vi "D-O Module (Main).vi"(7 "Name of Parent Panel":string="Main.vi", 9 "New Center Coords":T1={"Horizontal"=470, "Vertical"=200}, 10 "Config":variant, 11 "Main UI Message Queue":refnum<queue>) -> ()   [LabVIEW 2018, in "D-O Module.lvlib"]
doc: "This Continuous Measurement sample project is based on the Queued Message Handler template.\n\nThe Event Handling Loop generates messages based on user interface actions.\n\nThe Message Handling Loop processes messages generated by the Event Handling Loop, or by other messages. There are also Acquisition and Logging message handling loop subVIs, and a chart updating loop."
uses:
  D-O Module.lvlib
  support/Message Queue/Message Cluster.ctl
  <vilib>/Utility/miscctls.llb/LVPoint32TypeDef.ctl
  controls/UI Data.ctl
  controls/UI State.ctl
  D-O Module State Cluster.ctl
  D-O Module Config Cluster.ctl
  Valve Clusters.ctl
  D-O Module Settings Cluster.ctl
  D-O Device Settings Cluster.ctl
  VICI Electronic Actuator/VICI Electronic Actuator Settings.ctl
  Measure Instrument/State Enum.ctl
  D-O Module Display.ctl
  Sequencing/Squence Update Cluster.ctl
  support/Message Queue/Enqueue Message (Single).vi
  support/User Event - Stop/User Event - Stop.lvlib
  support/Support Library.lvlib
  support/Message Queue/Message Queue.lvlib
  Measure Instrument/D-O Module Engine.lvlib
  Measure Instrument/Feed Module Engine.lvlib
  Sequencing/Sequencing Library.lvlib
  D-O Settings Dialog.vi
  support/Command Log VIs/Command Logging.lvlib
  DIO Valve/VICI Electronic Actuator.lvlib
  Report Generation/Report Generation.lvlib
panel:
  out "Sequence Started":bool
  in  "Settings Button":bool
  out "ScanCode":i16
  out "Ring":u16(ring)=2
  out "Log File path":path
  out "Status":string
  in  "Exit":bool
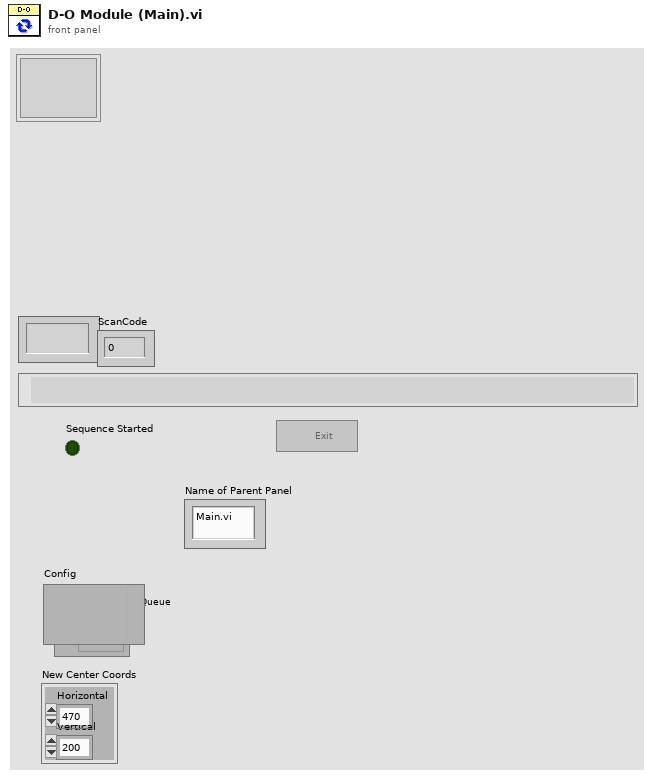
[diagram p1: front panel]
types:
  T1 = typedef "LVPoint32TypeDef.ctl" = cluster{"Horizontal":i32, "Vertical":i32}
  T2 = enum32{"Invalid", "Default", "Floating", "Floating/Auto-Hide", "Modal"}
  T3 = typedef "D-O Module.lvlib/D-O Module Config Cluster.ctl" = cluster{"GUID":string, "Drop Coords":T1, "Process Name":string, "User name":string, "Queue Name":string, "Settings":T4, "Load Count":i32}
  T4 = typedef "D-O Module.lvlib/Valve Clusters.ctl" = cluster{"Valve Settings":T5, "Valve Type":enum16{"Default", "Digital Output Valve", "VICI Electronic Actuator"}, "Time On (Sec)":dbl, "Time Off (Sec)":dbl, "Run?":bool}
  T5 = typedef "D-O Module.lvlib/D-O Module Settings Cluster.ctl" = cluster{"D-O Settings":T6, "VICI Electronic Actuator":T7}
  T6 = typedef "D-O Module.lvlib/D-O Device Settings Cluster.ctl" = cluster{"DAQmx Task Name":refnum<k21>, "Output Channel":u16, "Output Channel Names":string[]}
  T7 = typedef "VICI Electronic Actuator.lvlib/VICI Electronic Actuator Settings.ctl" = cluster{"VISA resource name":refnum<visa-resource-name>, "Mode":enum16{"Two Positions With Stops", "Two Positions Without Stops", "Mutiposition"}, "Simulated":bool}
  T8 = typedef "D-O Module.lvlib/D-O Module State Cluster.ctl" = cluster{"D-O Module Config":T3, "State":T9, "Start Time":timestamp, "Current Time":timestamp, "First Iteration":bool, "Data":cluster{"Valve State":T5}, "Process Name":string, "Queue Name":string, "Program On?":bool}
  T9 = typedef "Feed Module.lvlib/Feed Module Engine.lvlib/State Enum.ctl" = enum16{"Measuring", "Idle", "Paused"}
  T10 = typedef "UI State.ctl" = enum16{"Idle", "Acquiring and Logging", "Waiting for Exit", "Waiting for Exit (Acq Stopped)", "Waiting for Exit (Log Stopped)", "Waiting for Stop", "Waiting for Stop (Acq Stopped)", "Waiting for Stop (Log Stopped)"}
  T11 = typedef "UI Data.ctl" = cluster{"Start Ref":refnum<vi>, "Trigger Ref":refnum<vi>, "Stop Ref":refnum<vi>, "Settings Ref":refnum<vi>, "Status Ref":refnum<vi>, "Exit Ref":refnum<vi>, "Data Ref":refnum<vi>}
  T12 = typedef "D-O Module.lvlib/All Message Queues.ctl" = cluster{"Engine":refnum<queue>, "D-O UI":refnum<queue>, "D-O Engine":refnum<queue>, "D-O Display":refnum<queue>}
  T13 = typedef "Sequencing Library.lvlib/Squence Update Cluster.ctl" = cluster{"Auto?":bool, "Manual Entry":dbl, "Setpoint":dbl}
  T14 = enum8{"Enabled", "Disabled", "Disabled and Grayed Out"}
  T15 = typedef "D-O Module.lvlib/D-O Module Display.ctl" = cluster{"D-O State ":u16, "Cycle Period":dbl}
  T16 = cluster{"Shift":bool, "Ctrl":bool, "Alt":bool, "Cmd":bool, "Opt":bool}
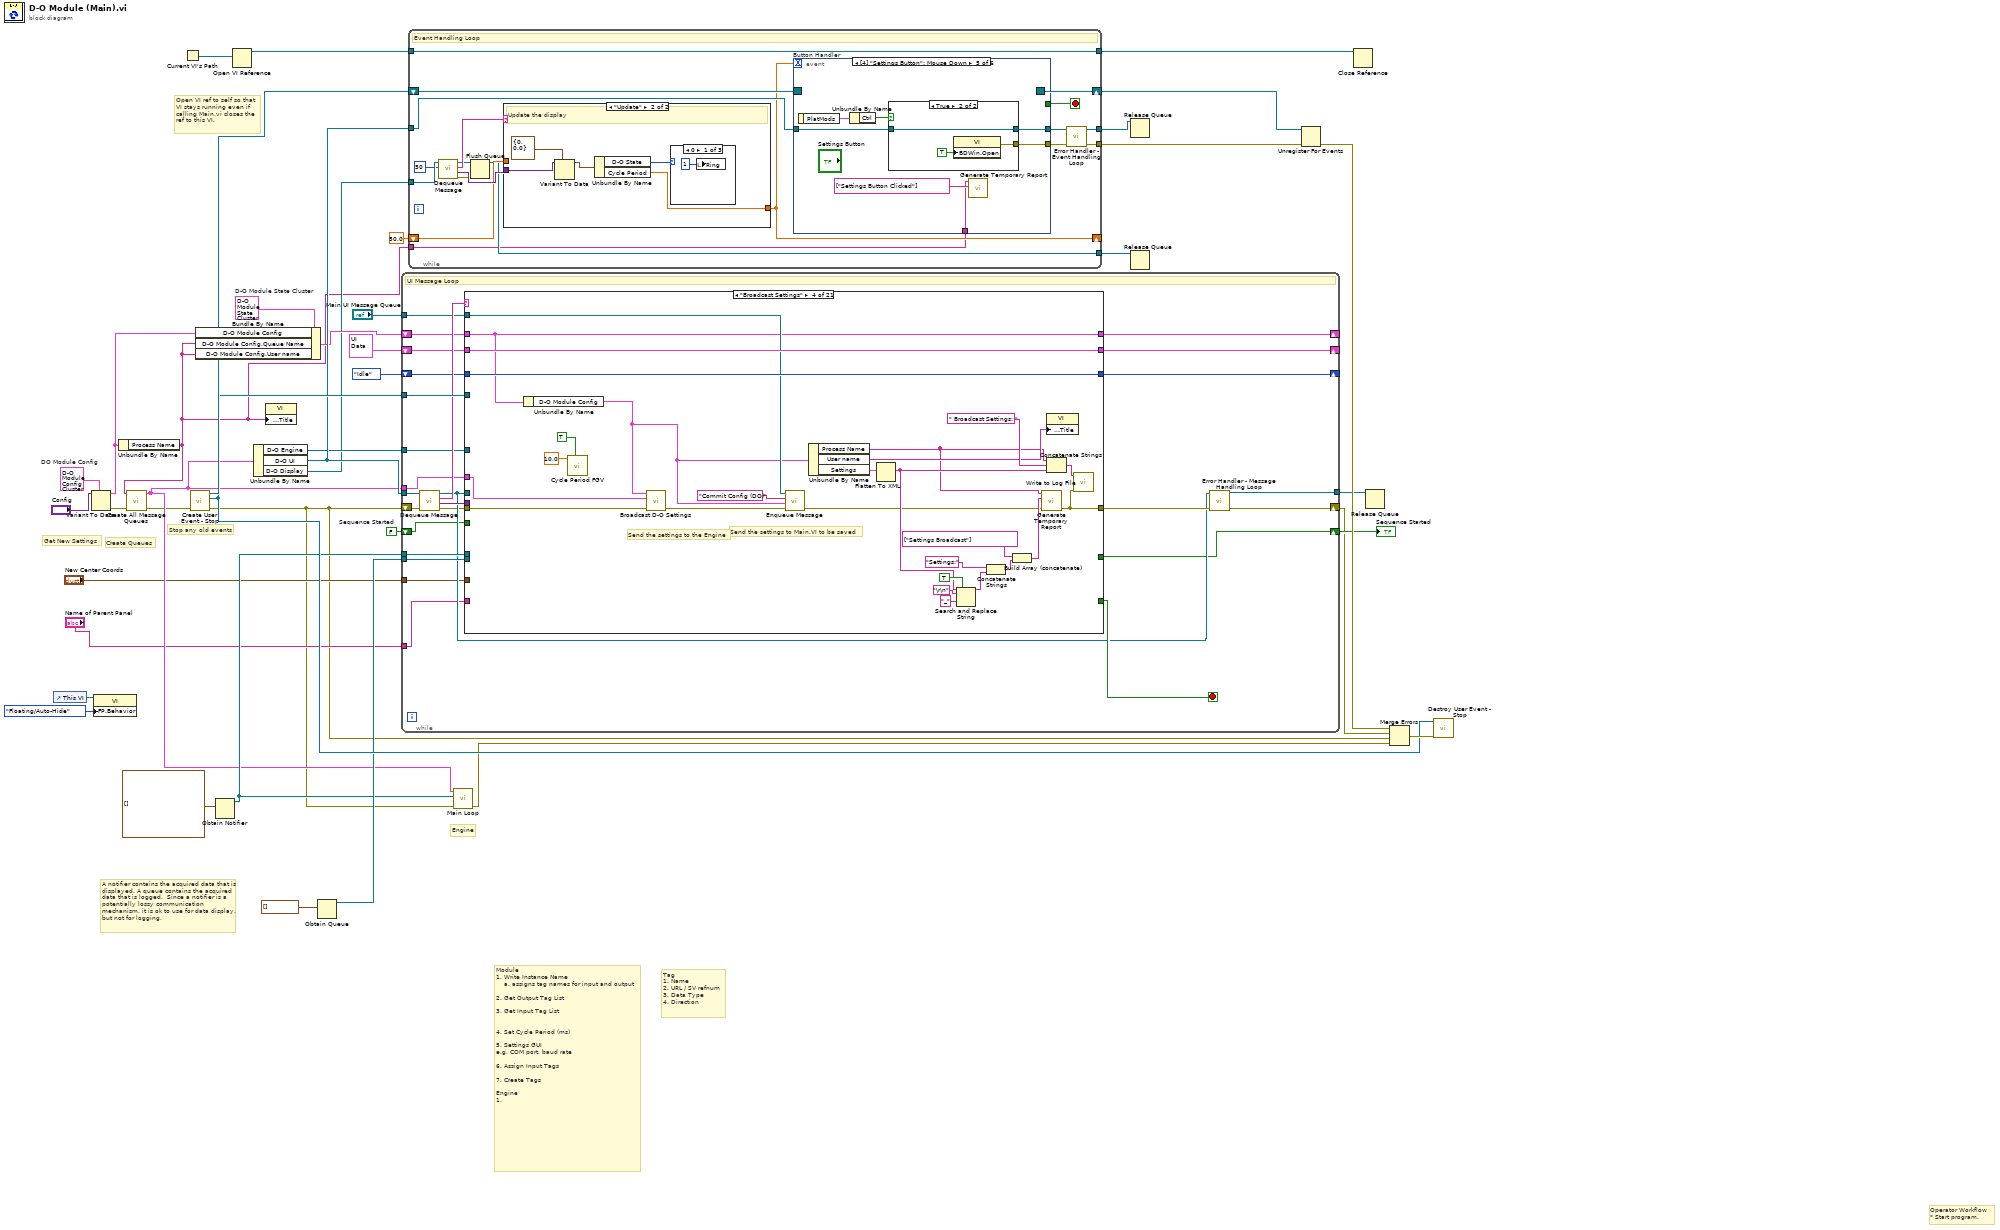
[diagram p0: block diagram]
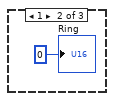
[diagram p3: hidden frame]
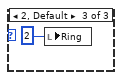
[diagram p4: hidden frame]
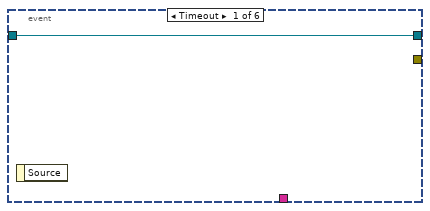
[diagram p5: hidden frame]
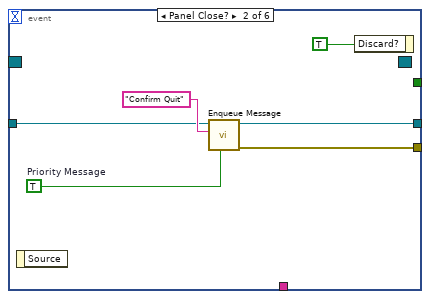
[diagram p6: hidden frame]
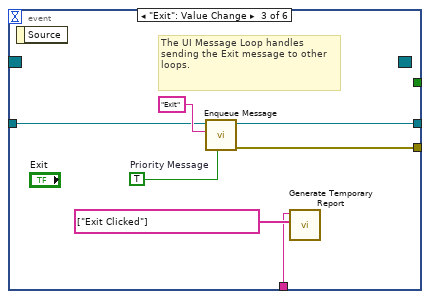
[diagram p7: hidden frame]
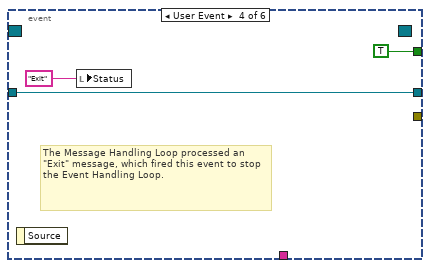
[diagram p8: hidden frame]
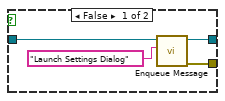
[diagram p9: hidden frame]
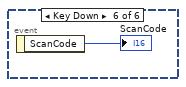
[diagram p10: hidden frame]
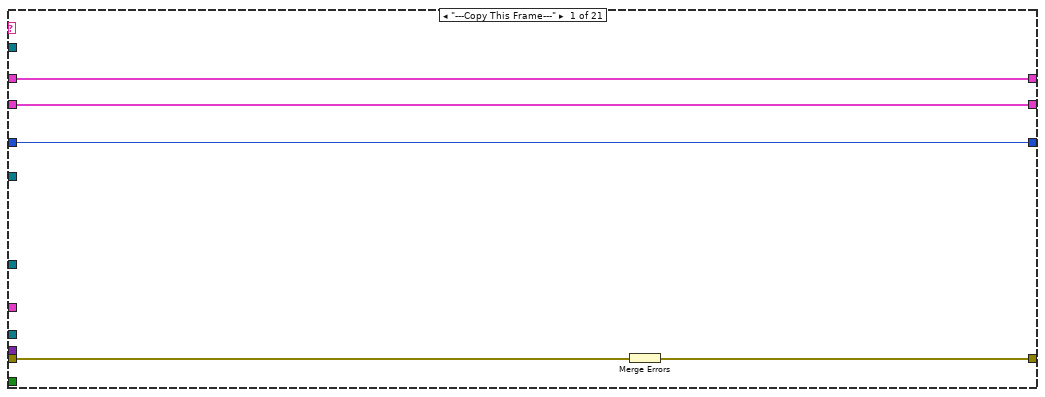
[diagram p11: hidden frame]
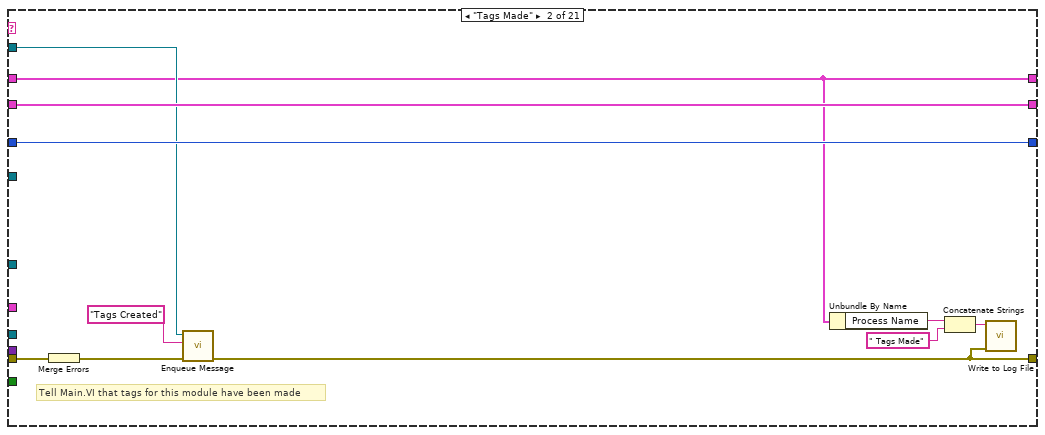
[diagram p12: hidden frame]
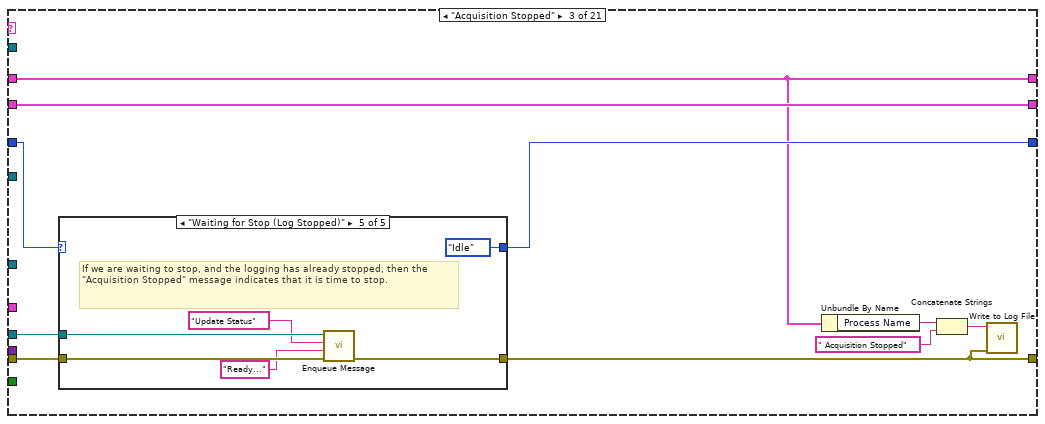
[diagram p13: hidden frame]
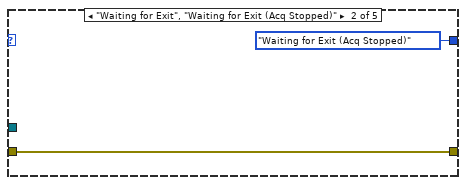
[diagram p15: hidden frame]
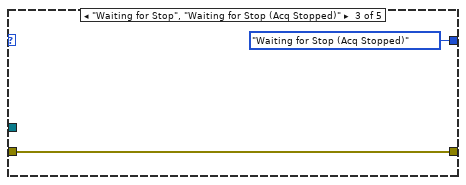
[diagram p16: hidden frame]
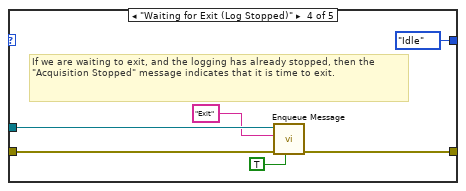
[diagram p17: hidden frame]
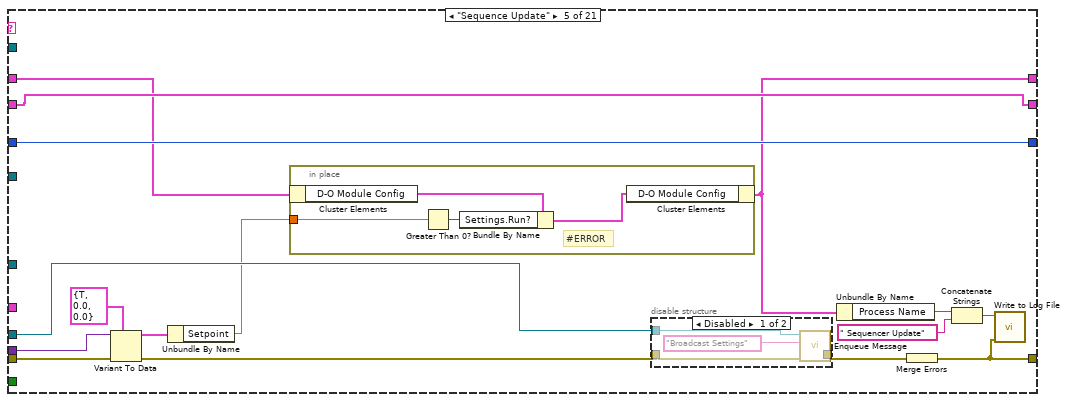
[diagram p18: hidden frame]
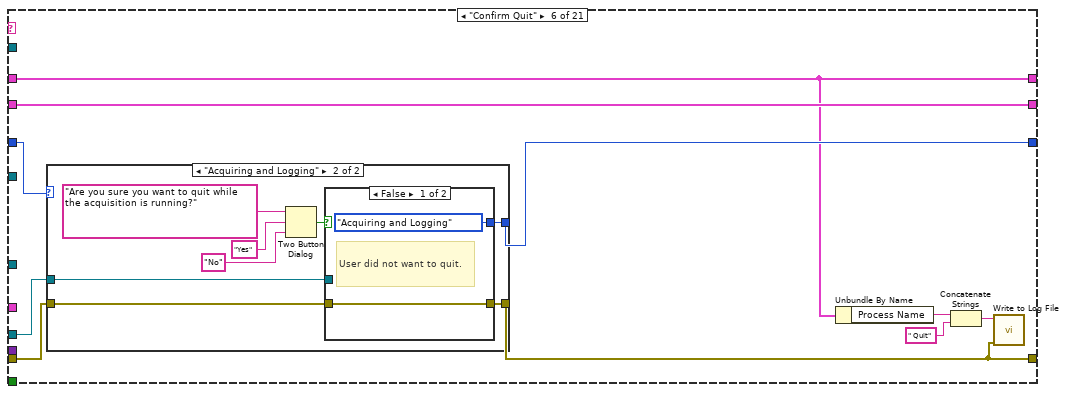
[diagram p20: hidden frame]
diagram:
  w14 = FALSE  # Sequence Started
  w13 = T3 {"GUID"="", "Drop Coords"={"Horizontal"=0, "Vertical"=0}, "Process Name"="", "User name"="", "Queue Name"="", "Settings"={"Valve Settings"={"D-O Settings"={"DAQmx Task Name"="", "Output Channel"=0, "Output Channel Names"=[]}, "VICI Electronic Actuator"={"VISA resource name"="", "Mode"=enum."Two Positions With Stops", "Simulated"=FALSE}}, "Valve Type"=enum."Default", "Time On (Sec)"=0.0, "Time Off (Sec)"=0.0, "Run?"=FALSE}, "Load Count"=0}  # DO Module Config
  w21 = T8 {"D-O Module Config"={"GUID"="", "Drop Coords"={"Horizontal"=0, "Vertical"=0}, "Process Name"="", "User name"="", "Queue Name"="", "Settings"={"Valve Settings"={"D-O Settings"={"DAQmx Task Name"="", "Output Channel"=0, "Output Channel Names"=[]}, "VICI Electronic Actuator"={"VISA resource name"="", "Mode"=enum."Two Positions With Stops", "Simulated"=FALSE}}, "Valve Type"=enum."Digital Output Valve", "Time On (Sec)"=0.0, "Time Off (Sec)"=0.0, "Run?"=FALSE}, "Load Count"=0}, "State"=enum."Idle", "Start Time"=timestamp(0 s since 1904-01-01), "Current Time"=timestamp(0 s since 1904-01-01), "First Iteration"=FALSE, "Data"={"Valve State"={"D-O Settings"={"DAQmx Task Name"="", "Output Channel"=0, "Output Channel Names"=[]}, "VICI Electronic Actuator"={"VISA resource name"="", "Mode"=enum."Two Positions With Stops", "Simulated"=FALSE}}}, "Process Name"="", "Queue Name"="", "Program On?"=FALSE}  # D-O Module State Cluster
  # "Stop any old events"
  # "Create Queues"
  # "Get New Settings"
  # "Open VI ref to self so that\nVI stays running even if\ncalling Main.vi closes the\nref to this VI."
  # "Engine"
  # "Operator Workflow\n* Start program."
  # "Module \n1. Write Instance Name\n    a. assigns tag names for input and output\n\n2. Get Output Tag List\n\n3. Get Input Tag List\n\n\n4. Set Cycle Period (ms)\n\n5. Settings GUI\ne.g. COM port, baud rate\n\n6. Assign Input Tags\n\n7. Create Tags\n\nEngine\n1."
  # "Tag\n1. Name\n2. URL / SV refnum\n3. Data Type\n4. Direction"
  # "A notifier contains the acquired data that is displayed. A queue contains the acquired data that is logged.  Since a notifier is a potentially lossy communication mechanism, it is ok to use for data display, but not for logging."
  n1 = control-ref of="This VI"() -> (w3:refnum<vi>)
  n2 = Variant To Data(type=w13, Variant="Config") -> (data=w12:T3, error out=w11:errorcluster)  [unwired: 1 in]
  n3 = property class="VI"(reference=w3, "FP.Behavior"=T2."Floating/Auto-Hide" ("Front Panel Window:Behavior")) -> ()  [unwired: 1 in, 2 out]
  n4 = Unbundle By Name(w12) -> ("Process Name"=w1:string)
  n5 = call "Create All Message Queues.vi"("error in (no error)"=w11, "Process Name"=w1) -> ("error out"=w10:errorcluster, "Message Queues"=w18:T12)  [unwired: 8 in]
  n6 = Current VI's Path() -> (path=w24:path)
  n7 = call "Create User Event - Stop.vi"("error in (no error)"=w10) -> ("error out"=w9:errorcluster, "User Event - Stop"=w38:refnum<user-event>, "Stop Event Registration Refnum"=w39:refnum<event-registration>)  [unwired: 8 in]
  n8 = Bundle By Name(cluster=w21, "D-O Module Config"=w12, "D-O Module Config.Queue Name"=w1, "D-O Module Config.User name"=w1) -> (w23:T8)
  n9 = Obtain Notifier(notification data type=waveform(dbl)[] []) -> (notifier out=w27:refnum<notifier>)  [unwired: 3 in, 2 out]
  n10 = Open VI Reference(vi path=w24) -> (vi reference=w25:refnum<vi>)  [unwired: 5 in, 1 out]
  n11 = Unbundle By Name(w18) -> ("D-O Engine"=w30:refnum<queue>, "D-O UI"=w34:refnum<queue>, "D-O Display"=w20:refnum<queue>)
  n12 = property class="VI"("Front Panel.Title"=w1) -> ()  [unwired: 2 in, 2 out]
  n13 = Obtain Queue(element data type=waveform(dbl)[] []) -> (queue out=w29:refnum<queue>)  [unwired: 4 in, 2 out]
  n14 = while {
    tunnel: w34 -> [w62]
    tunnel: w38 -> [w66]
    shift-right: [w56] -> w5
    shift-left: w9 -> [w65]
    shift-right: [w43] -> _
    shift-left: w23 -> [w50]
    shift-right: [w60] -> _
    shift-left: T11 {"Start Ref"=refnum, "Trigger Ref"=refnum, "Stop Ref"=refnum, "Settings Ref"=refnum, "Status Ref"=refnum, "Exit Ref"=refnum, "Data Ref"=refnum} ("Measurement UI Controls") -> [w61]
    tunnel: w27 -> [w59]
    tunnel: w29 -> [w58]
    shift-right: [w53] -> _
    shift-left: UI_State."Idle" ("UI State") -> [w54]
    tunnel: w30 -> [w52]
    tunnel: "Main UI Message Queue" -> [w49]
    tunnel: w18 -> [w48]
    tunnel: "New Center Coords" -> [w47]
    tunnel: "Name of Parent Panel" -> [w46]
    shift-right: [w45] -> w15
    shift-left: w14 -> [w44]
    tunnel: [w42] -> w4
    stop <- w67 stop-if-true
    # "UI Message Loop"
    n15 = call "Dequeue Message.vi"("error in (no error)"=w65, "Message Queue"=w62) -> ("error out"=w51:errorcluster, "Message Data"=w63:variant, "Message"=w64:string, "dup Message Queue"=w55:refnum<queue>)  [unwired: 6 in]
    n16 = case "Message Cases" shown="\"Broadcast Settings\"" w64 {
      selector: w64 -> [_ _ _ _ _ _ _ _ _ _ _ _ _ _ _ _ _ _ _ _ w507]
      tunnel: w55 -> [_ _ w89 _ w151 w170 _ w230 w245 w274 _ w308 w327 w333 w369 w400 _ _ w464 _ _]
      tunnel: w51 -> [w72 w83 w90 w135 w150 w169 w196 w211 w249 w278 w293 w303 w325 w335 w367 w399 w429 w439 w466 w499 _]
      tunnel: [w71 w77 w88 w113 w141 w164 w197 w202 w239 w251 w293 w298 w321 w334 w358 w388 w421 w444 w455 w500 w506] -> w57
      tunnel: [_ _ _ _ _ _ _ _ _ TRUE _ _ _ _ _ _ _ _ _ _ _] -> w67
      tunnel: w63 -> [_ _ _ _ w152 _ w199 _ w248 w262 _ _ _ _ _ _ _ _ _ w498 _]
      tunnel: w66 -> [_ _ _ _ _ _ _ _ _ w277 _ _ _ _ _ _ _ _ _ _ _]
      tunnel: w50 -> [w68 w73 w84 w132 w140 w163 w194 w209 w236 w255 w284 w294 w316 w332 w363 w395 w428 w440 w468 w489 w512]
      tunnel: w61 -> [w70 w82 w93 w138 w153 w172 w201 w227 w250 w275 w292 w304 w329 w338 w364 w396 w432 w449 w484 w495 w517]
      tunnel: [w70 w82 w93 w138 w153 w172 w201 w227 w250 w275 w291 w304 w329 w338 w364 w396 w432 w449 w484 w495 w517] -> w60
      tunnel: w59 -> [_ _ _ _ _ _ _ _ _ w273 _ _ _ _ _ _ _ _ _ _ _]
      tunnel: w58 -> [_ _ _ _ _ _ _ _ _ w269 _ _ _ _ _ _ _ _ _ _ _]
      tunnel: w54 -> [w69 w81 w92 w137 w154 w171 w195 w216 w240 _ _ _ w328 w337 _ _ _ _ w473 w490 w516]
      tunnel: [w69 w81 w91 w137 w154 w168 w195 w217 w240 UI_State."Idle" ("UI State") UI_State."Idle" ("UI State") UI_State."Idle" ("UI State") w328 w336 UI_State."Acquiring and Logging" ("UI State") UI_State."Acquiring and Logging" ("UI State") UI_State."Acquiring and Logging" ("UI State") UI_State."Acquiring and Logging" ("UI State") w474 w490 w516] -> w53
      tunnel: w52 -> [_ _ _ _ _ _ _ w215 _ w261 _ _ _ _ _ _ w430 w447 w472 _ _]
      tunnel: w49 -> [_ w78 _ w134 _ _ _ _ _ w263 _ _ _ _ _ _ _ _ _ _ _]
      tunnel: [w68 w73 w84 w132 w139 w163 w194 w206 w236 w255 w284 w294 w317 w332 w357 w385 w428 w440 w459 w489 w512] -> w43
      tunnel: w48 -> [_ _ _ w130 _ _ _ _ _ _ _ _ w323 _ _ _ _ _ _ _ _]
      tunnel: w47 -> [_ _ _ _ _ _ _ _ _ _ _ w301 _ _ _ _ _ _ _ _ _]
      tunnel: w46 -> [_ _ _ _ _ _ _ _ _ _ _ w300 _ _ _ _ _ _ _ _ _]
      tunnel: [_ _ _ _ _ _ _ _ _ _ _ _ _ _ _ w393 _ _ _ _ _] -> w45
      tunnel: w44 -> [_ _ _ _ _ _ _ _ _ _ _ _ _ _ _ w389 _ _ _ _ _]
      frame "---Copy This Frame---" {
        # "Duplicate this frame when creating new messages.  Change this comment in the duplicated frame to describe this message."
        n17 = Merge Errors(w72) -> (w71:errorcluster)
      }
      frame "Tags Made" {
        # "Tell Main.VI that tags for this module have been made"
        # "Duplicate this frame when creating new messages.  Change this comment in the duplicated frame to describe this message."
        n18 = Merge Errors(w83) -> (w79:errorcluster)
        n19 = call-poly "Enqueue Message.vi"("error in (no error)"=w79, "Message"="Tags Created", "Message Queue"=w78) -> ("error out"=w77:errorcluster)  [unwired: 7 in, 1 out]
        n20 = Unbundle By Name(w73) -> ("Process Name"=w76:string)
        n21 = Concatenate Strings(w76, " Tags Made" ("text")) -> (w74:string)
        n22 = call "Write to Log File.vi"("error in"=w77, "text"=w74) -> ()  [unwired: 9 in, 1 out]
      }
      frame "Acquisition Stopped" {
        # "Logic for determining what action to take when the acquisition has stopped."
        n23 = case shown="\"Waiting for Stop (Log Stopped)\"" w92 {
          selector: w92 -> [w95 _ _ _ _]
          tunnel: [w95 UI_State."Waiting for Exit (Acq Stopped)" ("UI State") UI_State."Waiting for Stop (Acq Stopped)" ("UI State") UI_State."Idle" ("UI State") UI_State."Idle" ("UI State")] -> w91
          tunnel: w90 -> [w94 w96 w98 w104 w110]
          tunnel: [w94 w96 w98 w103 w109] -> w88
          tunnel: w89 -> [_ _ _ w102 w108]
          frame Default {
          }
          frame "Waiting for Exit", "Waiting for Exit (Acq Stopped)" {
          }
          frame "Waiting for Stop", "Waiting for Stop (Acq Stopped)" {
          }
          frame "Waiting for Exit (Log Stopped)" {
            # "If we are waiting to exit, and the logging has already stopped, then the \"Acquisition Stopped\" message indicates that it is time to exit."
            n24 = call-poly "Enqueue Message.vi"("Priority Message? (F)"=TRUE, "error in (no error)"=w104, "Message"="Exit", "Message Queue"=w102) -> ("error out"=w103:errorcluster)  [unwired: 6 in, 1 out]
          }
          frame "Waiting for Stop (Log Stopped)" {
            # "If we are waiting to stop, and the logging has already stopped, then the \"Acquisition Stopped\" message indicates that it is time to stop."
            n25 = call-poly "Enqueue Message.vi"("error in (no error)"=w110, "Message Data"="Ready..." ("Message"), "Message"="Update Status", "Message Queue"=w108) -> ("error out"=w109:errorcluster)  [unwired: 6 in, 1 out]
          }
        }
        n26 = Unbundle By Name(w84) -> ("Process Name"=w87:string)
        n27 = Concatenate Strings(w87, " Acquisition Stopped" ("text")) -> (w85:string)
        n28 = call "Write to Log File.vi"("error in"=w88, "text"=w85) -> ()  [unwired: 9 in, 1 out]
      }
      frame "Broadcast Settings" {
        # "Send the settings to Main.VI to be saved"
        # "Send the settings to the Engine"
        # "Send the 'Update Settings' message to the Logging and Acquisition message loops."
        n29 = Unbundle By Name(w132) -> ("D-O Module Config"=w126:T3)
        n30 = call "Cycle Period FGV.vi"("Write"=TRUE, "Cycle Period In (ms)"=10.0) -> ()  [unwired: 8 in, 2 out]
        n31 = call "Broadcast D-O Settings.vi"("error in (no error)"=w135, "Message Queues"=w130, "D-O Module Config"=w126) -> ("error out"=w133:errorcluster)  [unwired: 8 in]
        n32 = call-poly "Enqueue Message.vi"("error in (no error)"=w133, "Message Data"=w126, "Message"="Commit Config (DO)", "Message Queue"=w134) -> ("error out"=w114:errorcluster)  [unwired: 6 in, 1 out]
        n33 = Unbundle By Name(w126) -> ("Process Name"=w112:string, "User name"=w125:string, "Settings"=w117:T4)
        n34 = Flatten To XML(anything=w117) -> (xml string=w115:string)
        n35 = Search and Replace String(replace all?=TRUE ("replace all? (F)"), input string=w115, search string="\r\n", replace string="_" ("replace string (\"\")")) -> (result string=w116:string)  [unwired: 4 in, 3 out]
        n36 = Concatenate Strings("Settings:" ("string"), w116) -> (w123:string)
        n37 = Build Array (concatenate)(string[] ["Settings Broadcast"] ("Line of Events"), w123) -> (w118:string[])
        n38 = call "Generate Temporary Report.vi"("error in (no error)"=w114, "Line of Events"=w118, "Module Name"=w112) -> ("error out"=w113:errorcluster)  [unwired: 8 in]
        n39 = property class="VI"("Front Panel.Title"=w125) -> ()  [unwired: 2 in, 2 out]
        n40 = Concatenate Strings(w112, " Broadcast Settings: " ("text"), w115) -> (w127:string)
        n41 = call "Write to Log File.vi"("error in"=w113, "text"=w127) -> ()  [unwired: 9 in, 1 out]
      }
      frame "Sequence Update" {
        n42 = Variant To Data(error in=w150, type=T13 {"Auto?"=TRUE, "Manual Entry"=0.0, "Setpoint"=0.0} ("Cluster"), Variant=w152) -> (data=w148:T13, error out=w146:errorcluster)
        n43 = Unbundle By Name(w148) -> ("Setpoint"=w145:dbl)
        n44 = in-place {
          in-place-border: w145 -> [w161]
          # "#ERROR"
          n45 = in-place-cluster #1(w140) -> ("D-O Module Config"=w160:T3)
          n46 = Greater Than 0?(x=w161) -> (x > 0?=w162:bool)
          n47 = Bundle By Name(cluster=w160, "Settings.Run?"=w162) -> (w159:T3)
          n48 = in-place-cluster #1("D-O Module Config"=w159) -> (w139:T8)
        }
        n49 = disable-structure shown="Disabled" {
          disable-tunnel: w151 -> [w158 _]
          disable-tunnel: [w157 _] -> w147
          disable-tunnel: w146 -> [w155 _]
          frame Disabled {
            n50 = call-poly "Enqueue Message.vi"("error in (no error)"=w155, "Message"="Broadcast Settings", "Message Queue"=w158) -> ("error out"=w157:errorcluster)  [unwired: 7 in, 1 out]
          }
          frame Enabled {
          }
        }
        n51 = Unbundle By Name(w139) -> ("Process Name"=w144:string)
        n52 = Merge Errors(w147) -> (w141:errorcluster)
        n53 = Concatenate Strings(w144, " Sequencer Update" ("text")) -> (w142:string)
        n54 = call "Write to Log File.vi"("error in"=w141, "text"=w142) -> ()  [unwired: 9 in, 1 out]
      }
      frame "Confirm Quit" {
        # "Confirm Quit - Message that can confirm whether or not the user wants to exit the application."
        n55 = case shown="\"Acquiring and Logging\"" w171 {
          tunnel: w170 -> [w177 w183]
          tunnel: w169 -> [w176 w181]
          tunnel: [w173 w180] -> w164
          tunnel: [UI_State."Idle" ("UI State") w179] -> w168
          frame Default {
            # "If 'Confirm Quit' comes in while the system is idle, there is no need for a confirmation message."
            n56 = call-poly "Enqueue Message.vi"("Priority Message? (F)"=TRUE, "error in (no error)"=w176, "Message"="Exit", "Message Queue"=w177) -> ("error out"=w173:errorcluster)  [unwired: 6 in, 1 out]
          }
          frame "Acquiring and Logging" {
            n57 = Two Button Dialog(message="Are you sure you want to quit while the acquisition is running?" ("Confirm Quit Message"), 1:"No" ("No"), 2:"Yes" ("Yes")) -> (T button?=w182:bool)
            n58 = case shown="False" w182 {
              tunnel: w183 -> [_ w193]
              tunnel: w181 -> [w187 w192]
              tunnel: [w187 w191] -> w180
              tunnel: [UI_State."Acquiring and Logging" ("UI State") UI_State."Waiting for Exit" ("UI State")] -> w179
              frame False {
                # "User did not want to quit."
              }
              frame True {
                n59 = call-poly "Enqueue Message.vi"("error in (no error)"=w192, "Message"="Stop", "Message Queue"=w193) -> ("error out"=w191:errorcluster)  [unwired: 7 in, 1 out]
              }
            }
          }
        }
        n60 = Unbundle By Name(w163) -> ("Process Name"=w167:string)
        n61 = Concatenate Strings(w167, " Quit" ("text")) -> (w165:string)
        n62 = call "Write to Log File.vi"("error in"=w164, "text"=w165) -> ()  [unwired: 9 in, 1 out]
      }
      frame "Display Log File Path" {
        n63 = Variant To Data(error in=w196, type=path "", Variant=w199) -> (data=→"Log File path":path, error out=w197:errorcluster)
      }
      frame "E-Stop" {
        # "Pause the DO when E-Stop is sent"
        # "Message Acquisition and Logging loops to stop"
        # "Enable: Start, Exit, Settings\nDisable: Stop"
        # "Stop the pumps."
        n64 = Unbundle By Name(w227) -> ("Trigger Ref"=w218:refnum<vi>, "Stop Ref"=w219:refnum<vi>, "Start Ref"=w222:refnum<vi>, "Exit Ref"=w221:refnum<vi>, "Settings Ref"=w220:refnum<vi>)
        n65 = call-poly "Enqueue Message.vi"("error in (no error)"=w211, "Message Data"="Ready..." ("Ready..."), "Message"="Update Status", "Message Queue"=w230) -> ("error out"=w213:errorcluster)  [unwired: 6 in, 1 out]
        n66 = Build Array(w222, w221, w220) -> (w225:refnum<vi>[])
        n67 = Build Array(w218, w219) -> (w224:refnum<vi>[])
        n68 = call-poly "Enqueue Message.vi"("error in (no error)"=w213, "Message"="Pause", "Message Queue"=w215) -> ("error out"=w212:errorcluster)  [unwired: 7 in, 1 out]
        n69 = call "Set Enable State on Multiple Controls.vi"("Enable?"=FALSE, "Controls"=w224) -> ()  [unwired: 10 in]
        n70 = call "Set Enable State on Multiple Controls.vi"("Enable?"=TRUE, "Controls"=w225) -> ()  [unwired: 10 in]
        n71 = case shown="Default" w216 {
          selector: w216 -> [_ w232]
          tunnel: [UI_State."Waiting for Stop" ("UI State") w232] -> w217
          frame Default {
          }
          frame "Waiting for Exit" {
          }
        }
        n72 = Merge Errors(w212) -> (w203:errorcluster)
        n73 = Bundle By Name(cluster=w209, "State"=State_Enum."Idle") -> (w206:T8)
        n74 = Unbundle By Name(w206) -> ("Process Name"=w204:string)
        n75 = call "Generate Temporary Report.vi"("error in (no error)"=w203, "Line of Events"=string[] ["E-STOP"], "Module Name"=w204) -> ("error out"=w202:errorcluster)  [unwired: 8 in]
        n76 = Concatenate Strings(w204, " E-STOP" ("text")) -> (w207:string)
        n77 = call "Write to Log File.vi"("error in"=w202, "text"=w207) -> ()  [unwired: 9 in, 1 out]
      }
      frame "Error" {
        # "Error - Check the error message data and respond accordingly. This message is sent by the \"Error Handler\" VIs at the end of each loop in this application."
        n78 = Variant To Data(error in=w249, type=errorcluster {"status"=FALSE, "code"=0, "source"=""} ("error out"), Variant=w248) -> (data=w246:errorcluster, error out=w242:errorcluster)
        n79 = call <vilib>:"Simple Error Handler.vi"("error in (no error)"=w246) -> ()  [unwired: 4 in, 5 out]
        n80 = call-poly "Enqueue Message.vi"("Priority Message? (F)"=TRUE, "Message"="Exit", "Message Queue"=w245) -> ("error out"=w241:errorcluster)  [unwired: 7 in, 1 out]
        n81 = Merge Errors(w241, w242) -> (w239:errorcluster)
        n82 = Unbundle By Name(w236) -> ("Process Name"=w238:string)
        n83 = call <vilib>:"General Error Handler.vi"("error in (no error)"=w239) -> ("message"=w234:string, "error out"=w233:errorcluster)  [unwired: 10 in, 3 out]
        n84 = Concatenate Strings(w238, " Error: " ("text"), w234) -> (w237:string)
        n85 = call "Write to Log File.vi"("error in"=w233, "text"=w237) -> ()  [unwired: 9 in, 1 out]
      }
      frame "Exit" {
        w266 = TRUE  # Delete Module?
        # "Stop DO Engine then Close it"
        # "Don't check the error outs. The acquisition and logging queues may have already been released."
        # "Close references owned by the Main VI."
        # "Stop the VI"
        # "Exit - Fire the User Event to stop the Event Handling Loop.  Also send Exit messages to the Acquisition and Logging loops."
        n86 = Release Queue(queue=w274, error in (no error)=w278) -> (error out=w272:errorcluster)  [unwired: 1 in, 2 out]
        n87 = call "Fire User Event - Stop.vi"("User Event - Stop"=w277) -> ("error out"=w276:errorcluster)  [unwired: 10 in]
        n88 = Release Notifier(notifier=w273, error in (no error)=w272) -> (error out=w271:errorcluster)  [unwired: 1 in, 2 out]
        n89 = Release Queue(queue=w269, error in (no error)=w271) -> (error out=w270:errorcluster)  [unwired: 1 in, 2 out]
        n90 = call-poly "Enqueue Message.vi"("Message"="Stop", "Message Queue"=w261) -> ("dup Message Queue"=w259:refnum<queue>)  [unwired: 8 in, 1 out]
        n91 = Variant To Data(type=w266, Variant=w262) -> (data=w265:bool, error out=w267:errorcluster)  [unwired: 1 in]
        n92 = Select(t=w266, s=w267, f=w265) -> (s? t:f=w264:bool)
        n93 = call-poly "Enqueue Message.vi"("Message"="Exit", "Message Queue"=w259) -> ()  [unwired: 8 in, 2 out]
        n94 = case "Don't enqueue Delete Module if opening campaign because it\nwill already have been deleted and new config loaded and we create\na race condition." shown="True" w264 {
          tunnel: w263 -> [_ w282]
          tunnel: w255 -> [_ w281]
          frame False {
          }
          frame True {
            n95 = Unbundle By Name(w281) -> ("D-O Module Config.GUID"=w280:string)
            n96 = call-poly "Enqueue Message.vi"("Message Data"=w280, "Message"="Delete Module", "Message Queue"=w282) -> ()  [unwired: 7 in, 2 out]
          }
        }
        n97 = Merge Errors(w276, w270) -> (w252:errorcluster)
        n98 = Unbundle By Name(w255) -> ("Process Name"=w253:string)
        n99 = Concatenate Strings(w253, " Exit" ("text")) -> (w256:string)
        n100 = call "Generate Temporary Report.vi"("error in (no error)"=w252, "Line of Events"=string[] ["Exited"], "Module Name"=w253) -> ("error out"=w251:errorcluster)  [unwired: 8 in]
        n101 = call "Write to Log File.vi"("error in"=w251, "text"=w256) -> ()  [unwired: 9 in, 1 out]
      }
      frame "Init UI Refs" {
        # "Enable: Start, Exit, Settings\nDisable: Stop"
        # "Init UI Refs - Store control references for UI controls.  Also enable/disable controls appropriately."
        n102 = property class="VI"("Front Panel.Closeable"=TRUE ("Front Panel Window:Closeable")) -> ()  [unwired: 2 in, 2 out]
        n103 = control-ref of="Status"() -> (w289:refnum<vi>)
        n104 = control-ref of="Exit"() -> (w286:refnum<vi>)
        n105 = Bundle By Name(cluster=w292, "Status Ref"=w289, "Exit Ref"=w286) -> (w291:T11)
        n106 = Build Array(w286) -> (w288:refnum<vi>[])
        n107 = call "Set Enable State on Multiple Controls.vi"("Enable?"=TRUE, "Controls"=w288) -> ()  [unwired: 10 in]
      }
      frame "Initialize" {
        # "Initialize - Get configuration settings, then message the UI to initialize, and broadcast the settings to the other message loops."
        n108 = Unbundle By Name(w294) -> ("Process Name"=w299:string)
        n109 = property class="VI" props=["FP.State"]() -> (reference out=w302:refnum<vi>)  [unwired: 2 in, 2 out]
        n110 = call-poly "Enqueue Message.vi"("error in (no error)"=w303, "Message"="Init UI Refs", "Message Queue"=w308) -> ("error out"=w306:errorcluster, "dup Message Queue"=w307:refnum<queue>)  [unwired: 7 in]
        n111 = call "Make Child and Move.vi"("Process Name"=w299, "Name of Parent Panel"=w300, "New Center Coords"=w301, "VI in"=w302) -> ()  [unwired: 8 in]
        n112 = call-poly "Enqueue Message.vi"("error in (no error)"=w306, "Message"="Broadcast Settings", "Message Queue"=w307) -> ("error out"=w314:errorcluster, "dup Message Queue"=w313:refnum<queue>)  [unwired: 7 in]
        n113 = call-poly "Enqueue Message.vi"("error in (no error)"=w314, "Message Data"="Ready..." ("Ready..."), "Message"="Update Status", "Message Queue"=w313) -> ("error out"=w298:errorcluster)  [unwired: 6 in, 1 out]
        n114 = Unbundle By Name(w294) -> ("Process Name"=w297:string)
        n115 = Concatenate Strings(w297, " Initialize" ("text")) -> (w295:string)
        n116 = call "Write to Log File.vi"("error in"=w298, "text"=w295) -> ()  [unwired: 9 in, 1 out]
      }
      frame "Launch Settings Dialog" {
        # "Keep track of whether the Dialog has been opened."
        # "Launch the Settings Dialog when the user clicks the 'Settings' button."
        n117 = in-place {
          n118 = in-place-cluster #2(w316) -> ("D-O Module Config.Load Count"=w331:i32)
          n119 = Increment(x=w331) -> (x+1=w330:i32)
          n120 = in-place-cluster #2("D-O Module Config.Load Count"=w330) -> (w315:T8)
        }
        n121 = call-by-ref "?"("error in (no error)"=w325, "Message Queues"=w323, "D-O Module State Cluster In"=w315) -> ("error out"=w322:errorcluster, "D-O Module Config Out"=w324:T3)  [unwired: 7 in, 4 out]
        n122 = Bundle By Name(cluster=w316, "D-O Module Config"=w324) -> (w317:T8)
        n123 = call-poly "Enqueue Message.vi"("error in (no error)"=w322, "Message"="Broadcast Settings", "Message Queue"=w327) -> ("error out"=w321:errorcluster)  [unwired: 7 in, 1 out]
        n124 = Unbundle By Name(w317) -> ("Process Name"=w320:string)
        n125 = Concatenate Strings(w320, "Launch Settings Dialog" ("text")) -> (w318:string)
        n126 = call "Write to Log File.vi"("error in"=w321, "text"=w318) -> ()  [unwired: 9 in, 1 out]
      }
      frame "Logging Stopped" {
        # "Logic for determining what action to take when the logging has stopped."
        n127 = case shown="\"Waiting for Stop (Acq Stopped)\"" w337 {
          selector: w337 -> [w340 _ _ _ _]
          tunnel: [w340 UI_State."Waiting for Exit (Log Stopped)" ("UI State") UI_State."Waiting for Stop (Log Stopped)" ("UI State") UI_State."Idle" ("UI State") UI_State."Idle" ("UI State")] -> w336
          tunnel: w335 -> [w339 w341 w343 w349 w355]
          tunnel: [w339 w341 w343 w348 w354] -> w334
          tunnel: w333 -> [_ _ _ w347 w353]
          frame Default {
          }
          frame "Waiting for Exit", "Waiting for Exit (Log Stopped)" {
          }
          frame "Waiting for Stop", "Waiting for Stop (Log Stopped)" {
          }
          frame "Waiting for Exit (Acq Stopped)" {
            # "If we are waiting to exit, and the acquisition has already stopped, then the \"Logging Stopped\" message indicates that it is time to exit."
            n128 = call-poly "Enqueue Message.vi"("Priority Message? (F)"=TRUE, "error in (no error)"=w349, "Message"="Exit", "Message Queue"=w347) -> ("error out"=w348:errorcluster)  [unwired: 6 in, 1 out]
          }
          frame "Waiting for Stop (Acq Stopped)" {
            # "If we are waiting to stop, and the acquisition has already stopped, then the \"Logging Stopped\" message indicates that it is time to stop."
            n129 = call-poly "Enqueue Message.vi"("error in (no error)"=w355, "Message Data"="Ready..." ("Message"), "Message"="Update Status", "Message Queue"=w353) -> ("error out"=w354:errorcluster)  [unwired: 6 in, 1 out]
          }
        }
      }
      frame "Start" {
        # "Start the loops. In this case we could\n just do a straight start since there is \nonly one loop"
        # "Clear chart"
        # "Message Acquisition and Logging loops to start"
        # "Enable: Stop\nDisable: Start, Exit, Settings"
        # "Start - Enable/Disable buttons appropriately for an acquisition that has started, and update status display."
        n130 = Unbundle By Name(w364) -> ("Trigger Ref"=w375:refnum<vi>, "Stop Ref"=w376:refnum<vi>, "Start Ref"=w379:refnum<vi>, "Exit Ref"=w378:refnum<vi>, "Settings Ref"=w377:refnum<vi>, "Data Ref"=w366:refnum<vi>)
        n131 = property class="WFChart (strict)"(reference=w366, "History Data"=waveform(dbl)[][] []) -> ()  [unwired: 1 in, 2 out]
        n132 = Build Array(w379, w378, w377) -> (w382:refnum<vi>[])
        n133 = Build Array(w375, w376) -> (w381:refnum<vi>[])
        n134 = call-poly "Enqueue Message.vi"("error in (no error)"=w367, "Message"="Broadcast settings", "Message Queue"=w369) -> ("error out"=w370:errorcluster, "dup Message Queue"=w368:refnum<queue>)  [unwired: 7 in]
        n135 = call "Set Enable State on Multiple Controls.vi"("Enable?"=TRUE, "Controls"=w381) -> ()  [unwired: 10 in]
        n136 = call "Set Enable State on Multiple Controls.vi"("Enable?"=FALSE, "Controls"=w382) -> ()  [unwired: 10 in]
        n137 = call-poly "Enqueue Message.vi"("error in (no error)"=w370, "Message"="Start Loops", "Message Queue"=w368) -> ("error out"=w371:errorcluster)  [unwired: 7 in, 1 out]
        n138 = Merge Errors(w371) -> (w358:errorcluster)
        n139 = Bundle By Name(cluster=w363, "State"=State_Enum."Measuring") -> (w357:T8)
        n140 = Unbundle By Name(w357) -> ("Process Name"=w361:string)
        n141 = Concatenate Strings(w361, " Start" ("text")) -> (w359:string)
        n142 = call "Write to Log File.vi"("error in"=w358, "text"=w359) -> ()  [unwired: 9 in, 1 out]
      }
      frame "Sequence Start" {
        # "Clear chart"
        # "Message Acquisition and Logging loops to start"
        # "Enable: Stop\nDisable: Start, Exit, Settings"
        # "Start - Enable/Disable buttons appropriately for an acquisition that has started, and update status display."
        n143 = Unbundle By Name(w396) -> ("Trigger Ref"=w403:refnum<vi>, "Stop Ref"=w404:refnum<vi>, "Start Ref"=w407:refnum<vi>, "Exit Ref"=w406:refnum<vi>, "Settings Ref"=w405:refnum<vi>, "Data Ref"=w398:refnum<vi>)
        n144 = property class="WFChart (strict)"(reference=w398, "History Data"=waveform(dbl)[][] []) -> ()  [unwired: 1 in, 2 out]
        n145 = Build Array(w407, w406, w405) -> (w410:refnum<vi>[])
        n146 = Build Array(w403, w404) -> (w409:refnum<vi>[])
        n147 = call-poly "Enqueue Message.vi"("error in (no error)"=w399, "Message"="Broadcast settings", "Message Queue"=w400) -> ("error out"=w392:errorcluster, "dup Message Queue"=w391:refnum<queue>)  [unwired: 7 in]
        n148 = call "Set Enable State on Multiple Controls.vi"("Enable?"=TRUE, "Controls"=w409) -> ()  [unwired: 10 in]
        n149 = call "Set Enable State on Multiple Controls.vi"("Enable?"=FALSE, "Controls"=w410) -> ()  [unwired: 10 in]
        n150 = case shown="False" w389 {
          selector: w389 -> [_ w417]
          tunnel: [w416 w417] -> w393
          tunnel: w392 -> [w415 w418]
          tunnel: w391 -> [w413 _]
          tunnel: [w412 w418] -> w390
          frame False {
            w416 = TRUE  # Sequence Started
            # "Start the loops. In this case we could\n just do a straight start since there is \nonly one loop"
            # "Start the sequence loops"
            n151 = call-poly "Enqueue Message.vi"("error in (no error)"=w415, "Message"="Start Loops", "Message Queue"=w413) -> ("error out"=w412:errorcluster)  [unwired: 7 in, 1 out]
          }
          frame True {
            # "Sequence already started"
          }
        }
        n152 = Merge Errors(w390) -> (w388:errorcluster)
        n153 = Bundle By Name(cluster=w395, "State"=State_Enum."Measuring") -> (w385:T8)
        n154 = Unbundle By Name(w385) -> ("Process Name"=w387:string)
        n155 = Concatenate Strings(w387, " Sequence Start" ("text")) -> (w384:string)
        n156 = call "Write to Log File.vi"("error in"=w388, "text"=w384) -> ()  [unwired: 9 in, 1 out]
      }
      frame "Start Loops" {
        # "Start gets us going"
        # "Message Acquisition and Logging loops to start"
        # "Start - Enable/Disable buttons appropriately for an acquisition that has started, and update status display."
        n157 = Unbundle By Name(w428) -> ("D-O Module Config.Process Name"=w419:string, "D-O Module Config.Settings.Run?"=w423:bool)
        n158 = call-poly "Enqueue Message.vi"("error in (no error)"=w429, "Message Data"=w419, "Message"="Start", "Message Queue"=w430) -> ("error out"=w426:errorcluster, "dup Message Queue"=w424:refnum<queue>)  [unwired: 6 in]
        n159 = case shown="False" w423 {
          tunnel: w426 -> [w435 w437]
          tunnel: [w434 w437] -> w425
          tunnel: w424 -> [w433 _]
          frame False {
            # "If we are supposed to be paused we pause immediatly"
            n160 = call-poly "Enqueue Message.vi"("error in (no error)"=w435, "Message"="Pause", "Message Queue"=w433) -> ("error out"=w434:errorcluster)  [unwired: 7 in, 1 out]
          }
          frame True {
          }
        }
        n161 = Merge Errors(w425) -> (w422:errorcluster)
        n162 = call "Generate Temporary Report.vi"("error in (no error)"=w422, "Line of Events"=string[] ["Started"], "Module Name"=w419) -> ("error out"=w421:errorcluster)  [unwired: 8 in]
      }
      frame "Start Log" {
        # "Message Acquisition and Logging loops to start"
        # "Start - Enable/Disable buttons appropriately for an acquisition that has started, and update status display."
        n163 = Unbundle By Name(w440) -> ("D-O Module Config.Process Name"=w445:string)
        n164 = Build Array(w447) -> (w446:refnum<queue>[])
        n165 = for {
          tunnel: w439 -> [w453]
          tunnel: [w452] -> w438 mode=indexing
          tunnel: w446 -> [w451] mode=indexing
          tunnel: w445 -> [w450]
          n166 = call-poly "Enqueue Message.vi"("error in (no error)"=w453, "Message Data"=w450, "Message"="Start Log", "Message Queue"=w451) -> ("error out"=w452:errorcluster)  [unwired: 6 in, 1 out]
        }
        n167 = Merge Errors(w439, w438) -> (w444:errorcluster)
        n168 = Unbundle By Name(w440) -> ("Process Name"=w443:string)
        n169 = Concatenate Strings(w443, " Log Started" ("text")) -> (w441:string)
        n170 = call "Write to Log File.vi"("error in"=w444, "text"=w441) -> ()  [unwired: 9 in, 1 out]
      }
      frame "Stop" {
        # "Stop Pauses"
        # "Enable: Start, Exit, Settings\nDisable: Stop"
        # "Stop - Enable/Disable buttons appropriately for an acquisition that has stopped, and update status display."
        n171 = Unbundle By Name(w484) -> ("Trigger Ref"=w475:refnum<vi>, "Stop Ref"=w476:refnum<vi>, "Start Ref"=w479:refnum<vi>, "Exit Ref"=w478:refnum<vi>, "Settings Ref"=w477:refnum<vi>)
        n172 = call-poly "Enqueue Message.vi"("error in (no error)"=w466, "Message"="Broadcast settings", "Message Queue"=w464) -> ("error out"=w465:errorcluster, "dup Message Queue"=w463:refnum<queue>)  [unwired: 7 in]
        n173 = Build Array(w479, w478, w477) -> (w482:refnum<vi>[])
        n174 = Build Array(w475, w476) -> (w481:refnum<vi>[])
        n175 = call-poly "Enqueue Message.vi"("error in (no error)"=w465, "Message Data"="Ready..." ("Ready..."), "Message"="Update Status", "Message Queue"=w463) -> ("error out"=w471:errorcluster)  [unwired: 6 in, 1 out]
        n176 = call "Set Enable State on Multiple Controls.vi"("Enable?"=FALSE, "Controls"=w481) -> ()  [unwired: 10 in]
        n177 = call "Set Enable State on Multiple Controls.vi"("Enable?"=TRUE, "Controls"=w482) -> ()  [unwired: 10 in]
        n178 = call-poly "Enqueue Message.vi"("error in (no error)"=w471, "Message"="Pause", "Message Queue"=w472) -> ("error out"=w469:errorcluster)  [unwired: 7 in, 1 out]
        n179 = case shown="\"Waiting for Exit\"" w473 {
          selector: w473 -> [_ w488]
          tunnel: [UI_State."Waiting for Stop" ("UI State") w488] -> w474
          frame Default {
          }
          frame "Waiting for Exit" {
          }
        }
        n180 = Merge Errors(w469) -> (w456:errorcluster)
        n181 = Bundle By Name(cluster=w468, "State"=State_Enum."Paused") -> (w459:T8)
        n182 = Unbundle By Name(w459) -> ("Process Name"=w457:string)
        n183 = Concatenate Strings(w457, " Stopped" ("text")) -> (w460:string)
        n184 = call "Generate Temporary Report.vi"("error in (no error)"=w456, "Line of Events"=string[] ["Stopped"], "Module Name"=w457) -> ("error out"=w455:errorcluster)  [unwired: 8 in]
        n185 = call "Write to Log File.vi"("error in"=w455, "text"=w460) -> ()  [unwired: 9 in, 1 out]
      }
      frame "Update Status" {
        # "Update Display - Convert the message data to a string to display in the Status indicator."
        n186 = Variant To Data(error in=w499, type="", Variant=w498) -> (data=w492:string, error out=w496:errorcluster)
        "Status" <- w492
        n187 = Unbundle By Name(w495) -> ("Trigger Ref"=w491:refnum<vi>, "Stop Ref"=w494:refnum<vi>)
        n188 = property class="Bool"(reference=w494) -> ("DisabledEnum"=w493:T14)  [unwired: 1 in, 2 out]
        n189 = case shown="\"Enabled\"" w493 {
          tunnel: w492 -> [w503 _]
          tunnel: w491 -> [w504 _]
          frame "Enabled" {
            # "Disable the Force Trigger only while we are logging."
            n190 = Build Array(w504) -> (w505:refnum<vi>[])
            n191 = Not Equal?(x="Logging" ("Logging"), y=w503) -> (x != y?=w501:bool)
            n192 = call "Set Enable State on Multiple Controls.vi"("Enable?"=w501, "Controls"=w505) -> ()  [unwired: 10 in]
          }
          frame "Disabled", Default {
          }
        }
        n193 = Merge Errors(w496) -> (w500:errorcluster)
      }
      frame Default {
        # "'Default' case only runs if there is a message that isn't defined in any of the other cases.  Output a programming error."
        n194 = Concatenate Strings("The invalid message string " ("string"), w507, " was received in D-O Main." ("string")) -> (w508:string)
        n195 = Bundle By Name(cluster=errorcluster {"status"=TRUE, "code"=1, "source"=""} ("error constant"), "source"=w508) -> (w506:errorcluster)
        n196 = Unbundle By Name(w512) -> ("Process Name"=w515:string)
        n197 = Concatenate Strings(w515, " Invalid Message " ("text"), w507) -> (w513:string)
        n198 = call "Write to Log File.vi"("error in"=w506, "text"=w513) -> ()  [unwired: 9 in, 1 out]
      }
    }
    n199 = call "Error Handler - Message Handling Loop.vi"("error in (no error)"=w57, "Message Queue"=w55) -> ("dup error in"=w56:errorcluster, "dup Message Queue"=w42:refnum<queue>)  [unwired: 8 in]
  }
  "Sequence Started" <- w15
  n200 = while {
    tunnel: w34 -> [w530]
    tunnel: [w532] -> w41
    shift-right: [w531] -> w36
    shift-left: w39 -> [w536]
    tunnel: [w529] -> w26
    tunnel: w25 -> [w529]
    tunnel: w20 -> [w528]
    shift-right: [w525] -> _
    shift-left: 50.0 ("Cycle Period") -> [w524]
    tunnel: [w520] -> w7
    tunnel: [w519] -> w6
    tunnel: w1 -> [w518]
    stop <- w535 stop-if-true
    # "Event Handling Loop"
    n201 = call "Dequeue Message.vi"("timeout in ms (-1)"=50, "Message Queue"=w528) -> ("error out"=w521:errorcluster, "Message Data"=w526:variant, "Message"=w527:string, "dup Message Queue"=w522:refnum<queue>)  [unwired: 6 in]
    n202 = Flush Queue(queue=w522, error in (no error)=w521) -> (queue out=w519:refnum<queue>)  [unwired: 2 out]
    n203 = case shown="\"Update\"" w527 {
      tunnel: w526 -> [_ w542]
      tunnel: [w537 w538] -> w525
      tunnel: w524 -> [w537 _]
      frame "False", Default {
      }
      frame "Update" {
        # "Update the display"
        n204 = Variant To Data(type=T15 {"D-O State "=0, "Cycle Period"=0.0} ("FM Display"), Variant=w542) -> (data=w541:T15)  [unwired: 1 in, 1 out]
        n205 = Unbundle By Name(w541) -> ("D-O State"=w540:u16, "Cycle Period"=w538:dbl)
        n206 = case shown="0" w540 {
          frame 0 {
            n207 = local write "Ring"(u16 1 ("Ring")) -> ()
          }
          frame 1 {
            "Ring" <- u16 0 ("Ring")
          }
          frame 2, Default {
            n208 = local write "Ring"(u16 2 ("Ring")) -> ()
          }
        }
      }
    }
    n209 = event "Button Handler" shown="[4] \"Settings Button\": Mouse Down" {
      selector: w536 -> [_ _ _ _ _ _]
      dyn-events: [_ _ _ _ _ _] -> w531
      timeout: w525 -> [_ _ _ _ _ _]
      tunnel: [_ _ _ TRUE ("Discard?") _ _] -> w535
      tunnel: w530 -> [w546 w549 w556 w560 w567 _]
      tunnel: [_ w547 w559 _ w569 _] -> w533
      tunnel: [w546 w548 w555 w560 w568 _] -> w534
      tunnel: w518 -> [_ _ w553 _ w563 _]
      event Timeout {
        n210 = event-data() -> ()  [unwired: 1 in, 1 out]
      }
      event Panel Close? {
        w550 = TRUE  # Priority Message
        n211 = event-data() -> ()  [unwired: 1 in, 1 out]
        n212 = call-poly "Enqueue Message.vi"("Priority Message? (F)"=w550, "Message"="Confirm Quit", "Message Queue"=w549) -> ("error out"=w547:errorcluster, "dup Message Queue"=w548:refnum<queue>)  [unwired: 7 in]
        n213 = event-data("Discard?"=TRUE) -> ()  [unwired: 1 in, 1 out]
      }
      event "Exit": Value Change {
        w557 = TRUE  # Priority Message
        # "The UI Message Loop handles sending the Exit message to other loops."
        n214 = event-data() -> ()  [unwired: 1 in, 1 out]
        n215 = call-poly "Enqueue Message.vi"("Priority Message? (F)"=w557, "Message"="Exit", "Message Queue"=w556) -> ("error out"=w559:errorcluster, "dup Message Queue"=w555:refnum<queue>)  [unwired: 7 in]
        n216 = call "Generate Temporary Report.vi"("Line of Events"=string[] ["Exit Clicked"], "Module Name"=w553) -> ()  [unwired: 9 in, 1 out]
      }
      event User Event {
        # "The Message Handling Loop processed an \"Exit\" message, which fired this event to stop the Event Handling Loop."
        n217 = event-data() -> ()  [unwired: 1 in, 1 out]
        n218 = local write "Status"("Exit" ("Exit String")) -> ()
      }
      event "Settings Button": Mouse Down {
        n219 = event-data() -> ("PlatMods"=w566:T16)  [unwired: 1 in]
        n220 = Unbundle By Name(w566) -> ("Ctrl"=w565:bool)
        n221 = case shown="True" w565 {
          tunnel: [w573 w574] -> w569
          tunnel: [w572 w575] -> w568
          tunnel: w567 -> [w571 w575]
          frame False {
            n222 = call-poly "Enqueue Message.vi"("Message"="Launch Settings Dialog", "Message Queue"=w571) -> ("error out"=w573:errorcluster, "dup Message Queue"=w572:refnum<queue>)  [unwired: 8 in]
          }
          frame True {
            n223 = property class="VI"("BDWin.Open"=TRUE ("Block Diagram Window:Open")) -> (error out=w574:errorcluster)  [unwired: 2 in, 1 out]
          }
        }
        n224 = call "Generate Temporary Report.vi"("Line of Events"=string[] ["Settings Button Clicked"], "Module Name"=w563) -> ()  [unwired: 9 in, 1 out]
      }
      event Key Down {
        n225 = event-data() -> ("ScanCode"=→"ScanCode":i16)  [unwired: 1 in]
      }
    }
    n226 = call "Error Handler - Event Handling Loop.vi"("error in (no error)"=w533, "Message Queue"=w534) -> ("dup error in"=w532:errorcluster, "dup Message Queue"=w520:refnum<queue>)  [unwired: 8 in]
  }
  n227 = call "Main Loop.vi"("error in (no error)"=w9, "Chart Notifier"=w27, "Message Queues"=w18) -> ("error out"=w28:errorcluster)  [unwired: 8 in]
  n228 = Release Queue(queue=w7) -> ()  [unwired: 2 in, 3 out]
  n229 = Release Queue(queue=w6) -> ()  [unwired: 2 in, 3 out]
  n230 = Unregister For Events(event registration refnum=w36, error in=w41) -> (error out=w37:errorcluster)
  n231 = Close Reference(reference=w26) -> ()  [unwired: 1 in, 1 out]
  n232 = Release Queue(queue=w4) -> ()  [unwired: 2 in, 3 out]
  n233 = Merge Errors(w37, w5, w9, w28) -> (w40:errorcluster)
  n234 = call "Destroy User Event - Stop.vi"("error in (no error)"=w40, "User Event - Stop"=w38) -> ()  [unwired: 9 in, 1 out]
